vi "Populate Copy.vi"(8 "error in (no error)":errorcluster, 10 "Msg to Populate":refnum<class "Flex Msg.lvclass">, 11 "Source Msg":refnum<class "Flex Msg.lvclass">) -> (0 "error out":errorcluster, 2 "Populated Msg":refnum<class "Flex Msg.lvclass">)   [LabVIEW 2020, in "Msg.lvlib" / "Flex Msg.lvclass"]
doc: "Populate 'Msg to Populate' with data from 'Source Msg'. Use this VI if some private data is required for the operation of the message and cannot be written in any other way (as in nested message execution).\n\nThe default implementation does nothing."
uses:
  Flex Msg.lvclass
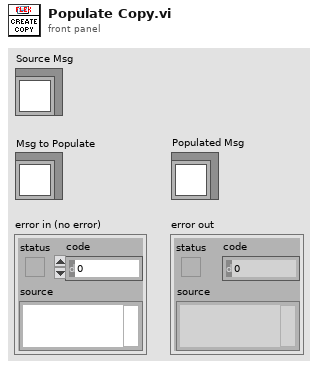
[diagram p1: front panel]
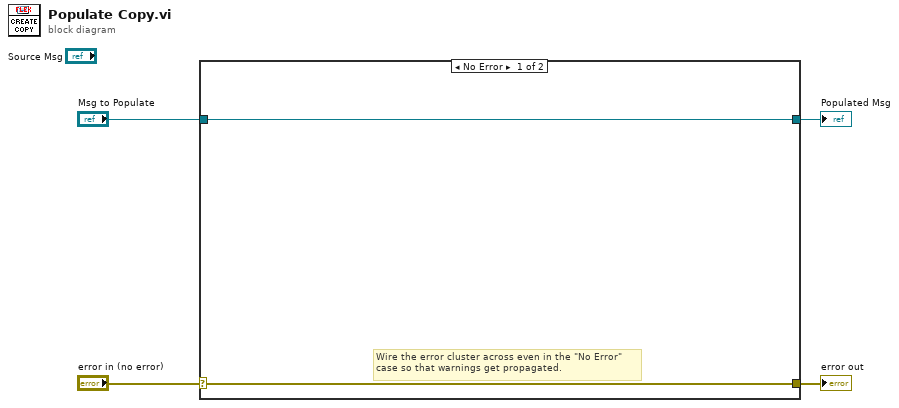
[diagram p0: block diagram]
diagram:
  n1 = case shown="No Error" "error in (no error)" {
    selector: "error in (no error)" -> [w5 w8]
    tunnel: [w5 w8] -> w3
    tunnel: [w6 w7] -> w1
    tunnel: "Msg to Populate" -> [w6 w7]
    frame No Error {
      # "Wire the error cluster across even in the \"No Error\"\ncase so that warnings get propagated."
    }
    frame Error {
    }
  }
  "error out" <- w3
  "Populated Msg" <- w1
